vi "setVoltageSpec.vi"(1 "Voltage":dbl min=0.0 max=5.0, 2 "DA_Spec":T1) -> ()   [LabVIEW 2011]
uses:
  DA_Spec.ctl
panel:
  out "Numeric 2":dbl caption="Channel"
  out "Numeric":dbl caption="Card"
  out "Slot":u16
  # "Channel Index"
  # "Card Index"
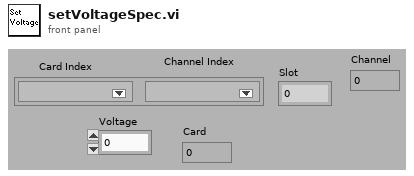
[diagram p1: front panel]
types:
  T1 = typedef "DA_Spec.ctl" = cluster{"Card Index":u16, "Channel Index":u16}
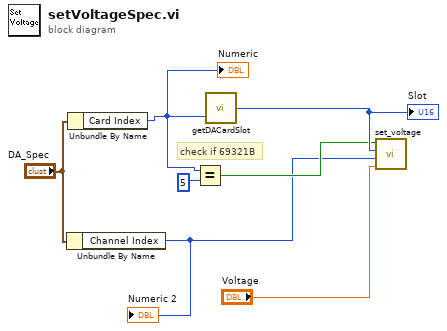
[diagram p0: block diagram]
diagram:
  # "check if 69321B"
  n1 = Unbundle By Name("DA_Spec") -> ("Channel Index"=w1:u16)
  "Numeric 2" <- w1
  n2 = Unbundle By Name("DA_Spec") -> ("Card Index"=w2:u16)
  "Numeric" <- w2
  n3 = Equal?(x=w2, y=u16 5) -> (x = y?=w3:bool)
  n4 = call "getDACardSlot.vi"("Card Index"=w2) -> ("Slot"=w4:u16)  [unwired: 1 in]
  "Slot" <- w4
  n5 = call "set_voltage.vi"("Voltage"="Voltage", "Channel Index"=w1, "Slot"=w4, "69321B?"=w3) -> ()  [unwired: 1 in]
